vi "Encoder Processing (SubVI).vi"(4 "Wheel Diameter":dbl, 5 "EncoderDevRef":T1, 7 "EncoderDevRef 2":T1) -> (0 "Distance (in) 2":dbl, 1 "Distance (in)":dbl, 2 "Encoder Rate R (deg/sec)":dbl, 3 "Encoder Rate  L(deg/sec) 2":dbl)   [LabVIEW 2015]
uses:
  <vilib>/Rock Robotics/WPI/Encoder/WPI_EncoderDevRef.ctl
  <vilib>/Rock Robotics/SystemInterfaces/Encoder/FPGA_EncoderIdx.ctl
  <vilib>/Rock Robotics/SystemInterfaces/Counter/FPGA_CounterCtrSystemIndex.ctl
  <vilib>/Rock Robotics/WPI/Encoder/WPI_EncoderType.ctl
  <vilib>/Rock Robotics/Network Tables/NT Read Boolean.vi
  <vilib>/Rock Robotics/Network Tables/NT Write Number.vi
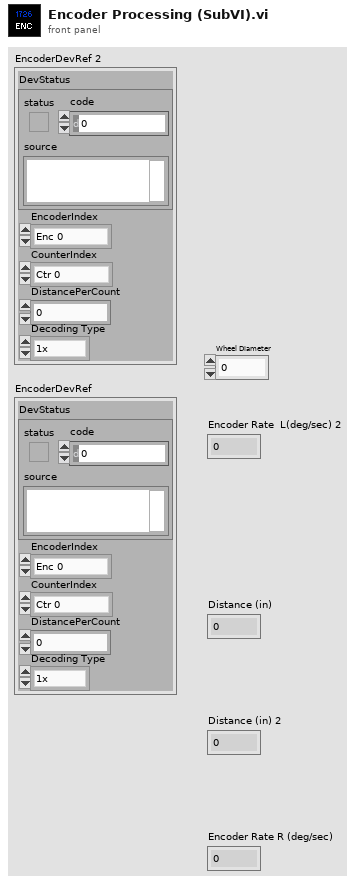
[diagram p1: front panel]
types:
  T1 = typedef "WPI_EncoderDevRef.ctl" = cluster{"DevStatus":errorcluster, "EncoderIndex":T2, "CounterIndex":T3, "DistancePerCount":dbl, "Decoding Type":T4}
  T2 = typedef "FPGA_EncoderIdx.ctl" = enum8{"Enc 0", "Enc 1", "Enc 2", "Enc 3", "Enc 4", "Enc 5", "Enc 6", "Enc 7", "Invalid"}
  T3 = typedef "FPGA_CounterCtrSystemIndex.ctl" = enum8{"Ctr 0", "Ctr 1", "Ctr 2", "Ctr 3", "Ctr 4", "Ctr 5", "Ctr 6", "Ctr 7", "Invalid"}
  T4 = typedef "WPI_EncoderType.ctl" = enum16{"1x", "2x", "4x"}
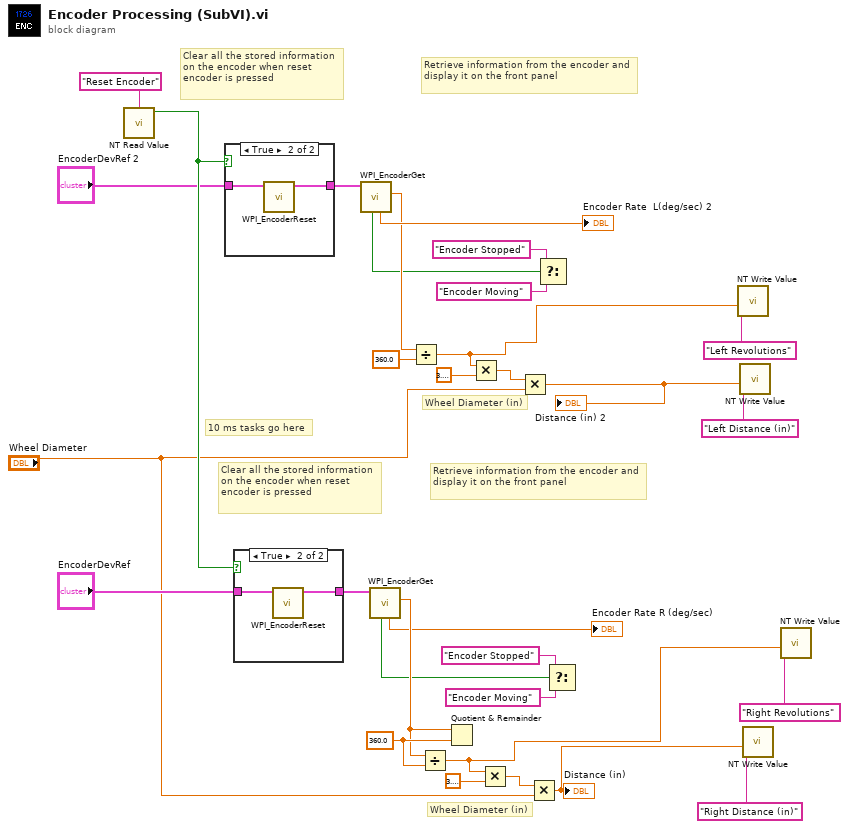
[diagram p0: block diagram]
diagram:
  w9 = 360.0 ("y")
  # "Wheel Diameter (in)"
  # "Wheel Diameter (in)"
  # "Retrieve information from the encoder and display it on the front panel"
  # "Clear all the stored information on the encoder when reset encoder is pressed"
  # "Retrieve information from the encoder and display it on the front panel"
  # "Clear all the stored information on the encoder when reset encoder is pressed"
  # "10 ms tasks go here"
  n1 = call-poly <vilib>:"NT Read Value.vi"("Name"="Reset Encoder") -> ("Boolean"=w31:bool)  [unwired: 9 in, 1 out]
  n2 = case shown="True" w31 {
    tunnel: "EncoderDevRef 2" -> [w32 w34]
    tunnel: [w32 w33] -> w12
    frame False {
    }
    frame True {
      n3 = call <vilib>:"WPI_EncoderReset.vi"("EncoderDevRef"=w34) -> ("EncoderDevRef"=w33:T1)  [unwired: 1 in, 9 out]
    }
  }
  n4 = case shown="True" w31 {
    tunnel: [w35 w37] -> w3
    tunnel: "EncoderDevRef" -> [w35 w36]
    frame False {
    }
    frame True {
      n5 = call <vilib>:"WPI_EncoderReset.vi"("EncoderDevRef"=w36) -> ("EncoderDevRef"=w37:T1)  [unwired: 1 in, 9 out]
    }
  }
  n6 = call <vilib>:"WPI_EncoderGet.vi"("EncoderDevRef"=w12) -> ("Distance"=w16:dbl, "Rate"=→"Encoder Rate  L(deg/sec) 2":dbl, "Stopped"=w13:bool)  [unwired: 1 in, 7 out]
  n7 = call <vilib>:"WPI_EncoderGet.vi"("EncoderDevRef"=w3) -> ("Distance"=w8:dbl, "Rate"=→"Encoder Rate R (deg/sec)":dbl, "Stopped"=w4:bool)  [unwired: 1 in, 7 out]
  n8 = Divide(x=w16, y=360.0) -> (x/y=w24:dbl)
  n9 = Divide(x=w8, y=w9) -> (x/y=w29:dbl)
  n10 = Quotient & Remainder(x=w8, y=w9) -> ()  [unwired: 2 out]
  n11 = Multiply(x=w24, y=3.141592653589793) -> (x*y=w18:dbl)
  n12 = Multiply(x=w29, y=3.141592653589793) -> (x*y=w11:dbl)
  n13 = Multiply(x=w18, y="Wheel Diameter") -> (x*y=w22:dbl)
  "Distance (in) 2" <- w22
  n14 = Multiply(x=w11, y="Wheel Diameter") -> (x*y=w27:dbl)
  "Distance (in)" <- w27
  n15 = Select(t="Encoder Stopped", s=w13, f="Encoder Moving") -> ()  [unwired: 1 out]
  n16 = Select(t="Encoder Stopped", s=w4, f="Encoder Moving") -> ()  [unwired: 1 out]
  n17 = call-poly <vilib>:"NT Write Value.vi"("Numeric"=w24, "Name"="Left Revolutions") -> ()  [unwired: 9 in, 1 out]
  n18 = call-poly <vilib>:"NT Write Value.vi"("Numeric"=w22, "Name"="Left Distance (in)") -> ()  [unwired: 9 in, 1 out]
  n19 = call-poly <vilib>:"NT Write Value.vi"("Numeric"=w27, "Name"="Right Distance (in)") -> ()  [unwired: 9 in, 1 out]
  n20 = call-poly <vilib>:"NT Write Value.vi"("Numeric"=w29, "Name"="Right Revolutions") -> ()  [unwired: 9 in, 1 out]
